vi "formula.vi"() -> ()   [LabVIEW 2018]
panel:
  in  "stop":bool
  out "X":dbl
  in  "b":dbl
  in  "a":dbl
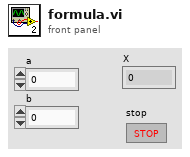
[diagram p1: front panel]
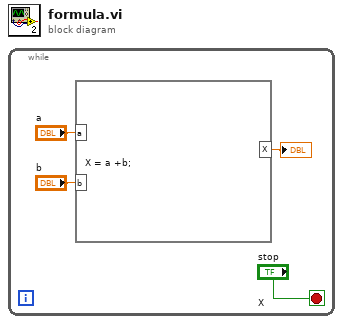
[diagram p0: block diagram]
diagram:
  n1 = while {
    stop <- "stop" stop-if-true
    n2 = formula code="X = a +b;"("a"="a", "b"="b") -> ("X"=→"X":dbl)
  }
